vi "Dequeue Broadcast Message by Message Cluster.vi"(8 "error in (no error)":errorcluster, 9 "Timeout (-1)":i32=-1, 10 "Message":T1, 11 "Event Registration Refnum":refnum<event-registration>) -> (0 "error out":errorcluster, 1 "Message Data":variant, 2 "Message":string, 3 "Event Registration Refnum Out":refnum<event-registration>, 4 "Timed Out?":bool)   [LabVIEW 2020, in "Broadcast Event Helpers.lvlib"]
doc: "Dequeue Broadcast messages filtering by message. The time out for this VI has an error margin of up to one time-out period in edge cases.\n\nThis VI is deperecated and a 1:1 replacement is available in the support directory. The event helper methods will be removed from TF.lvlib in a future release and should be replaced with the support library."
uses:
  Broadcast Event Helpers.lvlib
  Process/Protected/Broadcasting/Broadcast Message Cluster.ctl
  Broadcast Event Dequeuers/Broadcast Event Dequeuers.lvlib
  Process/Process.lvclass
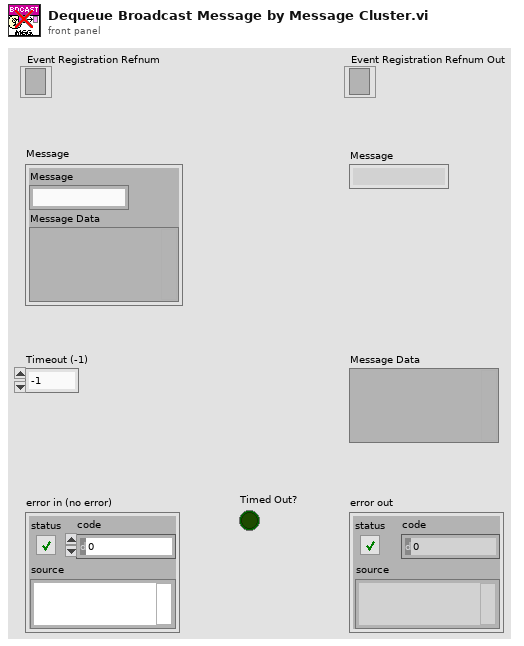
[diagram p1: front panel]
types:
  T1 = cluster{"Message":string, "Message Data":variant}
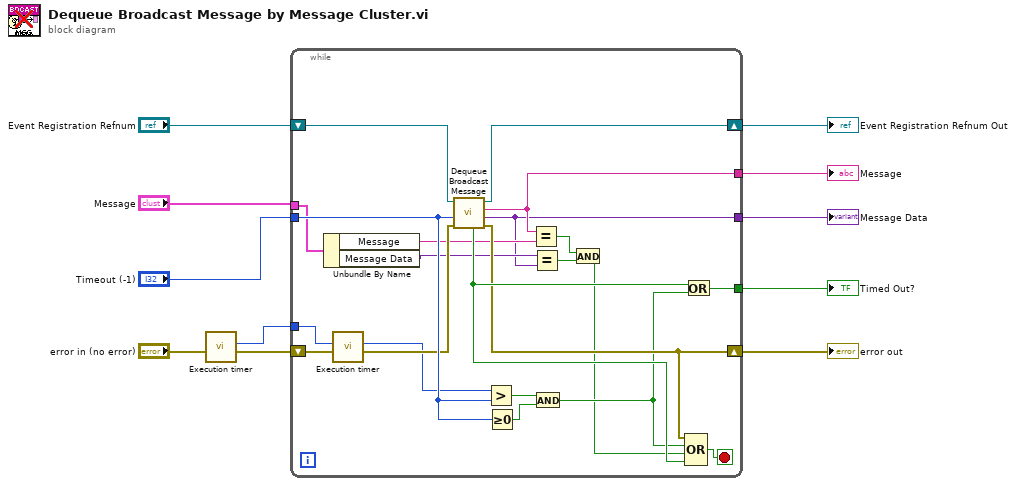
[diagram p0: block diagram]
diagram:
  n1 = call "Execution timer.vi"("error in (no error)"="error in (no error)") -> ("error out"=w3:errorcluster, "Current or Duration [ms]"=w2:u32)  [unwired: 9 in]
  n2 = while {
    tunnel: [w28] -> w7
    tunnel: [w14] -> w6
    tunnel: [w20] -> w5
    tunnel: "Timeout (-1)" -> [w25]
    shift-right: [w32] -> w10
    shift-left: "Event Registration Refnum" -> [w33]
    shift-right: [w21] -> w8
    shift-left: w3 -> [w31]
    tunnel: "Message" -> [w17]
    tunnel: w2 -> [w23]
    stop <- w30 stop-if-true
    n3 = Unbundle By Name(w17) -> ("Message"=w16:string, "Message Data"=w15:variant)
    n4 = call "Execution timer.vi"("error in (no error)"=w31, "millisecond timer value"=w23) -> ("error out"=w24:errorcluster, "Current or Duration [ms]"=w22:u32)  [unwired: 8 in]
    n5 = call "Dequeue Broadcast Message.vi"("error in (no error)"=w24, "Timeout (-1)"=w25, "Event Registration Refnum"=w33) -> ("error out"=w21:errorcluster, "Message Data"=w14:variant, "Message"=w28:string, "Event Registration Refnum Out"=w32:refnum<event-registration>, "Timed Out?"=w29:bool)  [unwired: 3 in, 1 out]
    n6 = Greater?(x=w22, y=w25) -> (0:w27:bool)
    n7 = Greater Or Equal To 0?(x=w25) -> (x >= 0?=w26:bool)
    n8 = Equal?(x=w28, y=w16) -> (x = y?=w18:bool)
    n9 = Equal?(x=w15, y=w14) -> (x = y?=w13:bool)
    n10 = And(x=w27, y=w26) -> (x .and. y?=w19:bool)
    n11 = And(x=w18, y=w13) -> (x .and. y?=w12:bool)
    n12 = Or(x=w29, y=w19) -> (x .or. y?=w20:bool)
    n13 = Compound Arithmetic op=OR(w21, w19, w12, w29) -> (w30:bool)
  }
  "Event Registration Refnum Out" <- w10
  "Message Data" <- w6
  "Message" <- w7
  "error out" <- w8
  "Timed Out?" <- w5
